vi "Pick_Freq.vi"(0 "time signal":waveform(dbl), 9 "RX frequency":dbl, 11 "sampling info":cluster{"Fs":dbl, "#s":dbl}={"Fs"=1000.0, "#s"=1000.0} {"Fs" format="%.2p"}) -> (4 "Mag":dbl, 6 "Phase":dbl, 8 "actual freq":dbl, 15 "signal out":waveform(dbl))   [LabVIEW 2020]
uses:
  <vilib>/Analysis/4window.llb/windowTd.ctl
  <vilib>/measure/maspectr.llb/FFT Spectrum (Mag-Phase) for 1 Chan.vi
  <vilib>/measure/NI_MAPro.lvlib
  <vilib>/measure/NI_MABase.lvlib
  <vilib>/Analysis/NI_AALPro.lvlib
panel:
  out "df":dbl
  in  "window":T1=1 items=["Rectangle"=0, "Hanning"=1, "Hamming"=2, "Blackman-Harris"=3, "Exact Blackman"=4, "Blackman"=5, "Flat Top"=6, "4 Term B-Harris "=7, "7 Term B-Harris"=8, "Low Sidelobe"=9, "Blackman Nuttall"=11, "Triangle"=30, "Bartlett-Hanning"=31, "Bohman"=32, "Parzen"=33, "Welch"=34, "Kaiser"=60, "Dolph-Chebyshev"=61, "Gaussian"=62]
  out "XY Graph":cluster{"Array":dbl[], "magnitude":dbl[]}(graph)
  out "Array":dbl[](array[numeric])
  out "index of Rx frequency":dbl
  # "Inputs:"
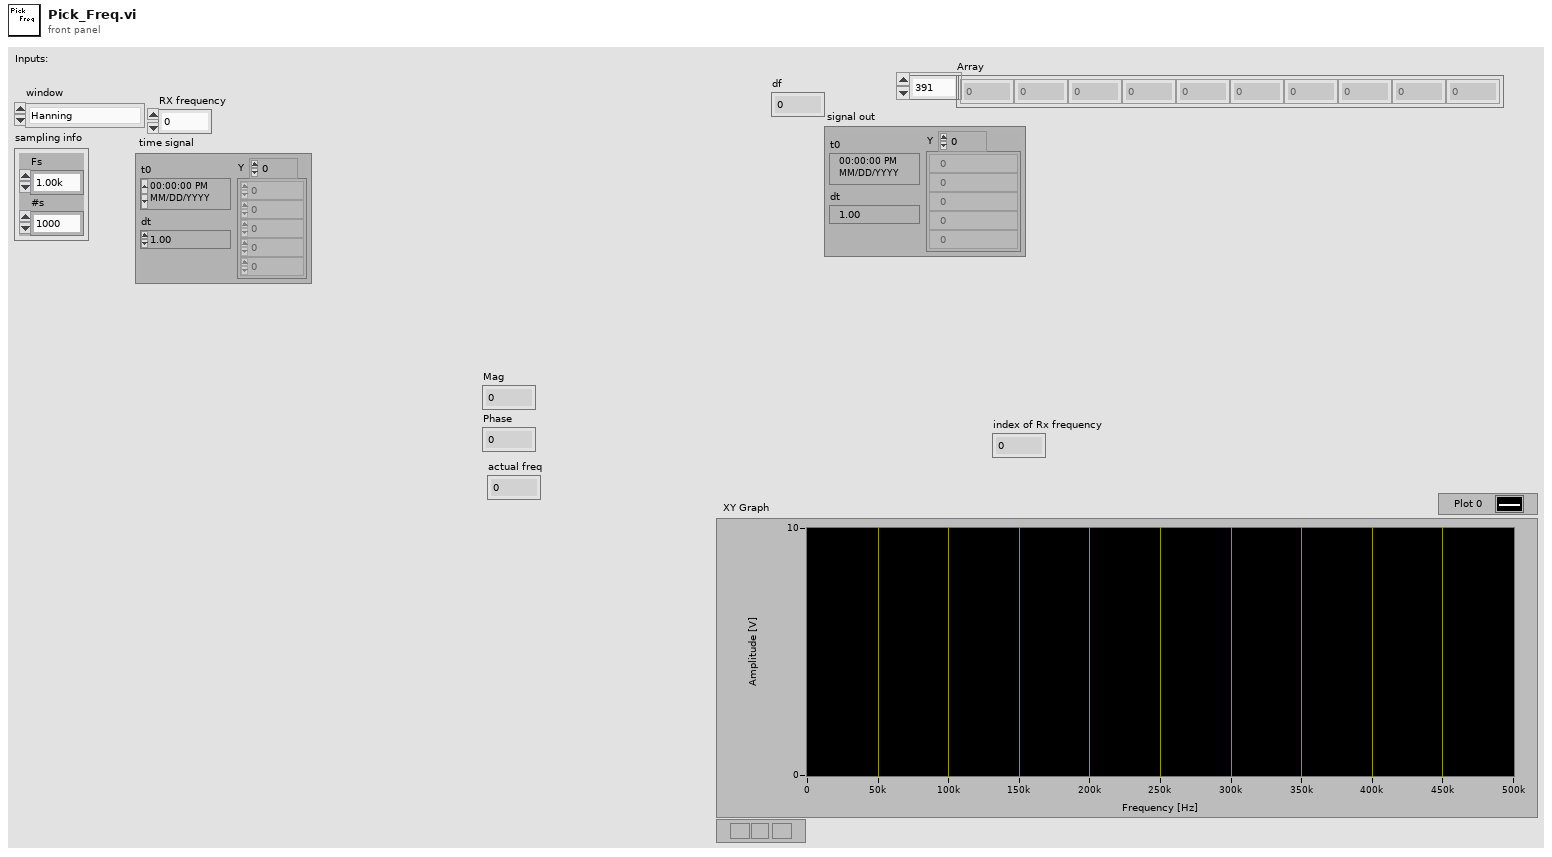
[diagram p1: front panel]
types:
  T1 = typedef "NI_AALPro.lvlib/windowTd.ctl" = u32
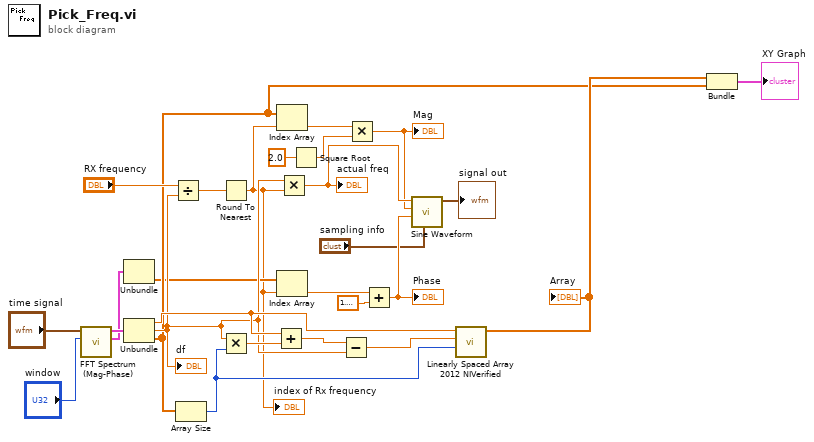
[diagram p0: block diagram]
diagram:
  n1 = call-poly <vilib>:"FFT Spectrum (Mag-Phase).vi"("window"="window", "time signal"="time signal") -> ("phase"=w15:cluster{"f0":dbl, "df":dbl, "phase":dbl[]}, "magnitude"=w16:cluster{"f0":dbl, "df":dbl, "magnitude":dbl[]})  [unwired: 5 in, 3 out]
  n2 = Unbundle(w15) -> ("phase"=w12:dbl[])  [unwired: 2 out]
  n3 = Unbundle(w16) -> ("f0"=w24:dbl, "df"=w19:dbl, "magnitude"=w13:dbl[])
  "df" <- w19
  n4 = Divide(x="RX frequency", y=w19) -> (x/y=w27:dbl)
  n5 = Array Size(array=w13) -> (size(s)=w22:i32)
  n6 = Round To Nearest(number=w27) -> (nearest integer value=w11:dbl)
  "index of Rx frequency" <- w11
  n7 = Multiply(x=w19, y=w22) -> (x*y=w25:dbl)
  n8 = Add(x=w24, y=w25) -> (x+y=w20:dbl)
  n9 = Index Array(array=w13, index=w11) -> (element=w10:dbl)
  n10 = Index Array(array=w12, index=w11) -> (element=w7:dbl)
  n11 = Multiply(x=w19, y=w11) -> (x*y=w5:dbl)
  "actual freq" <- w5
  n12 = Square Root(x=2.0) -> (sqrt(x)=w8:dbl)
  n13 = Subtract(x=w20, y=w19) -> (x-y=w21:dbl)
  n14 = Multiply(x=w10, y=w8) -> (x*y=w4:dbl)
  "Mag" <- w4
  n15 = Add(x=w7, y=1.5707963267948966) -> (x+y=w3:dbl)
  "Phase" <- w3
  n16 = call <vilib>:"Sine Waveform.vi"("sampling info"="sampling info", "phase"=w3, "amplitude"=w4, "frequency"=w5) -> ("signal out"=→"signal out":waveform(dbl))  [unwired: 6 in, 1 out]
  n17 = call "Linearly Spaced Array 2012 NIVerified.vi"("Number of Samples"=w22, "Maximum"=w21, "Minimum"=w24) -> ("Array"=w23:dbl[])  [unwired: 7 in, 1 out]
  "Array" <- w23
  n18 = Bundle("Array"=w23, "magnitude"=w13) -> (→"XY Graph":cluster{"Array":dbl[], "magnitude":dbl[]})  [unwired: 1 in]
